vi "ConsolidatedLimitSwitch.vi"(4 "Start at bottom?":bool=TRUE, 8 "CurrentLSValue":bool, 11 "CurrentInput":dbl) -> (2 "RelayValue":T1)   [LabVIEW 2013]
doc: "For use with coupled limit switches. Detects sign of input, maintains that, and blocks all input in that direction. Outputs relay signal. Requires LastSign and LastLSValue to be maintained by shift register in outside loop. Results unexpected when given 0 for CurrentInput."
uses:
  <vilib>/Rock Robotics/WPI/Relay/WPI_RelayValue.ctl
  LimitSwitchState.ctl
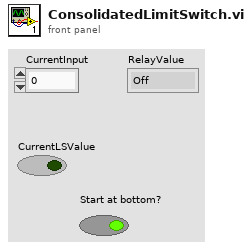
[diagram p1: front panel]
types:
  T1 = typedef "WPI_RelayValue.ctl" = enum16{"Off", "On", "Forward", "Reverse"}
  T2 = typedef "LimitSwitchState.ctl" = enum16{"Normal", "TopLS", "BottomLS", "Begin"}
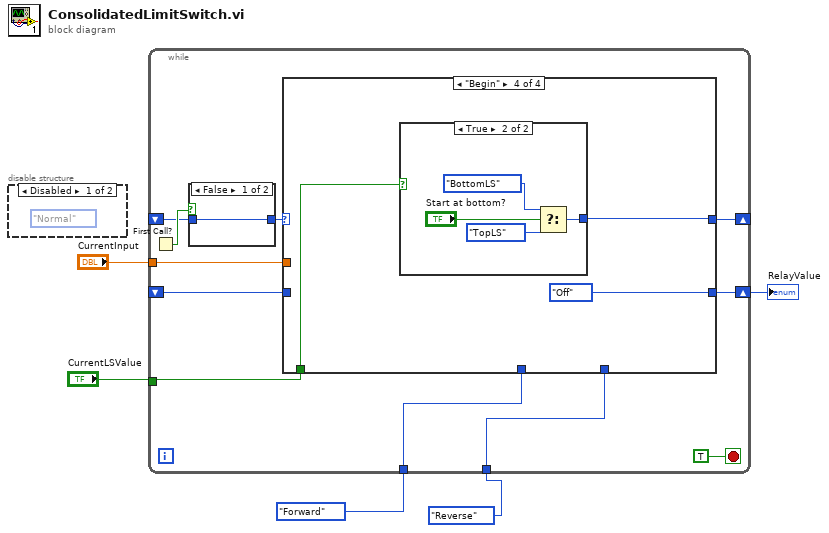
[diagram p0: block diagram]
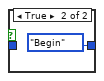
[diagram p3: hidden frame]
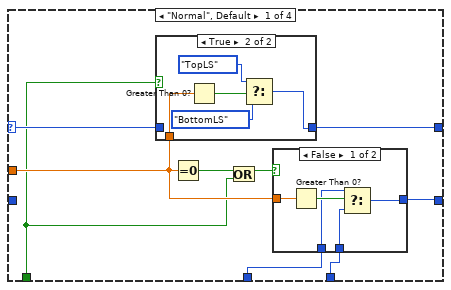
[diagram p4: hidden frame]
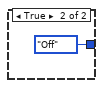
[diagram p5: hidden frame]
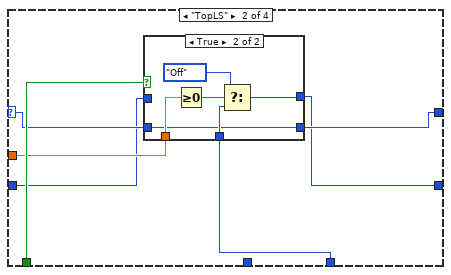
[diagram p7: hidden frame]
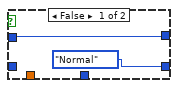
[diagram p8: hidden frame]
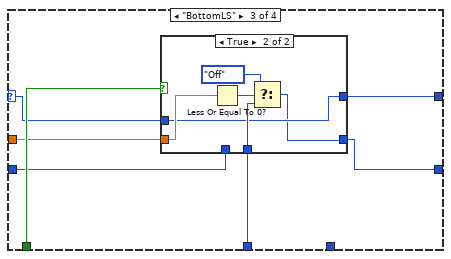
[diagram p9: hidden frame]
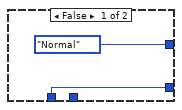
[diagram p10: hidden frame]
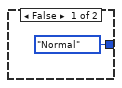
[diagram p11: hidden frame]
diagram:
  n1 = disable-structure shown="Disabled" {
    frame Disabled {
      (unwired) LimitSwitchState."Normal" ("f")
    }
    frame Enabled {
    }
  }
  n2 = while {
    tunnel: "CurrentInput" -> [w16]
    tunnel: "CurrentLSValue" -> [w15]
    tunnel: WPI_RelayValue."Reverse" ("f") -> [w14]
    tunnel: WPI_RelayValue."Forward" ("f") -> [w13]
    shift-right: [w11] -> _
    shift-left: _ -> [w9]
    shift-right: [w7] -> w3
    shift-left: _ -> [w6]
    stop <- TRUE stop-if-true
    n3 = First Call?() -> (First Call?: T/F=w10:bool)
    n4 = case shown="False" w10 {
      tunnel: [w17 LimitSwitchState."Begin" ("f")] -> w8
      tunnel: w9 -> [w17 _]
      frame False {
      }
      frame True {
      }
    }
    n5 = case shown="\"Begin\"" w8 {
      selector: w8 -> [w27 w45 w60 _]
      tunnel: w16 -> [w24 w44 w58 _]
      tunnel: w15 -> [w19 w46 w61 w70]
      tunnel: w14 -> [w22 w42 _ _]
      tunnel: w13 -> [w23 _ w57 _]
      tunnel: [w26 w43 w59 w72] -> w11
      tunnel: [w21 w41 w56 WPI_RelayValue."Off" ("f")] -> w7
      tunnel: w6 -> [_ w40 w55 _]
      frame "Normal", Default {
        n6 = case shown="True" w19 {
          tunnel: w27 -> [w34 _]
          tunnel: [w34 w37] -> w26
          tunnel: w24 -> [_ w38]
          frame False {
          }
          frame True {
            n7 = Greater Than 0?(x=w38) -> (x > 0?=w39:bool)
            n8 = Select(t=LimitSwitchState."TopLS" ("f"), s=w39, f=LimitSwitchState."BottomLS") -> (s? t:f=w37:T2)
          }
        }
        n9 = Equal To 0?(x=w24) -> (x = 0?=w25:bool)
        n10 = Or(x=w25, y=w19) -> (x .or. y?=w20:bool)
        n11 = case shown="False" w20 {
          tunnel: w24 -> [w32 _]
          tunnel: w23 -> [w30 _]
          tunnel: w22 -> [w29 _]
          tunnel: [w28 WPI_RelayValue."Off" ("f")] -> w21
          frame False {
            n12 = Greater Than 0?(x=w32) -> (x > 0?=w31:bool)
            n13 = Select(t=w30, s=w31, f=w29) -> (s? t:f=w28:T1)
          }
          frame True {
          }
        }
      }
      frame "TopLS" {
        n14 = case shown="True" w46 {
          tunnel: w45 -> [_ w51]
          tunnel: [LimitSwitchState."Normal" ("f") w51] -> w43
          tunnel: w44 -> [_ w53]
          tunnel: w42 -> [_ w52]
          tunnel: [w47 w49] -> w41
          tunnel: w40 -> [w47 _]
          frame False {
          }
          frame True {
            n15 = Greater Or Equal To 0?(x=w53) -> (x >= 0?=w54:bool)
            n16 = Select(t=WPI_RelayValue."Off", s=w54, f=w52) -> (s? t:f=w49:T1)
          }
        }
      }
      frame "BottomLS" {
        n17 = case shown="True" w61 {
          tunnel: w60 -> [_ w66]
          tunnel: [LimitSwitchState."Normal" ("f") w66] -> w59
          tunnel: w58 -> [_ w68]
          tunnel: w57 -> [_ w67]
          tunnel: [w62 w64] -> w56
          tunnel: w55 -> [w62 _]
          frame False {
          }
          frame True {
            n18 = Less Or Equal To 0?(x=w68) -> (x <= 0?=w69:bool)
            n19 = Select(t=WPI_RelayValue."Off", s=w69, f=w67) -> (s? t:f=w64:T1)
          }
        }
      }
      frame "Begin" {
        n20 = case shown="True" w70 {
          tunnel: [LimitSwitchState."Normal" ("f") w75] -> w72
          frame False {
          }
          frame True {
            n21 = Select(t=LimitSwitchState."BottomLS" ("f"), s="Start at bottom?", f=LimitSwitchState."TopLS") -> (s? t:f=w75:T2)
          }
        }
      }
    }
  }
  "RelayValue" <- w3
